vi "Calculadora con todo.vi"() -> ()   [LabVIEW 2020]
panel:
  in  "stop":bool
  in  "FUNCIONES":T1(ring)
  out "RESULTADO":dbl
  in  "NUM 2":dbl
  in  "NUM 1":dbl
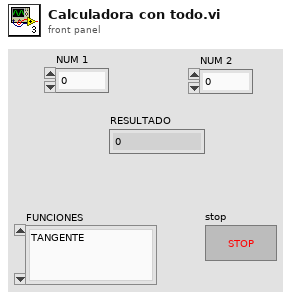
[diagram p1: front panel]
types:
  T1 = enum16{"TANGENTE", "COSENO", "SENO", "EXPONENCIAL", "CONVERSION GRADOS A RADIANES", "RAIZ CUADRADA", "DIVISION", "MULTIPLICACION", "RESTA", "SUMA"}
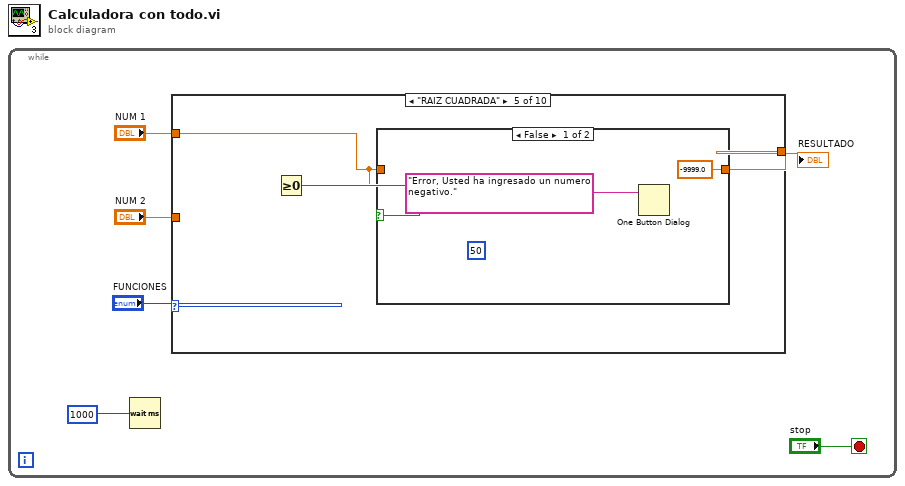
[diagram p0: block diagram]
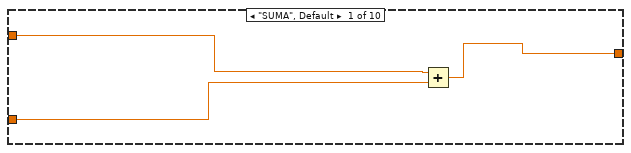
[diagram p2: hidden frame]
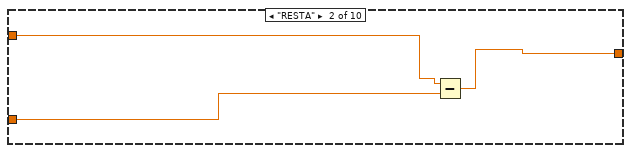
[diagram p3: hidden frame]
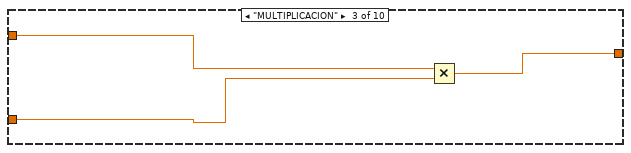
[diagram p4: hidden frame]
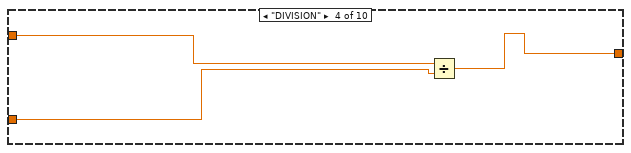
[diagram p5: hidden frame]
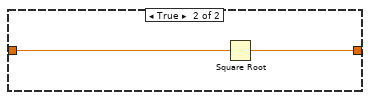
[diagram p6: hidden frame]
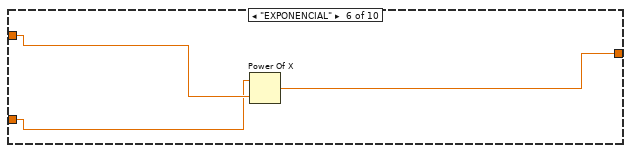
[diagram p7: hidden frame]
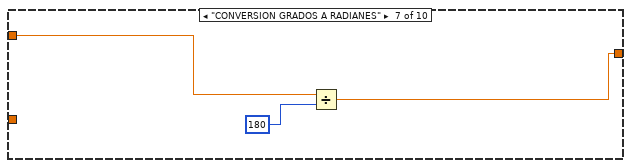
[diagram p8: hidden frame]
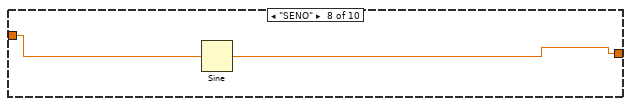
[diagram p9: hidden frame]
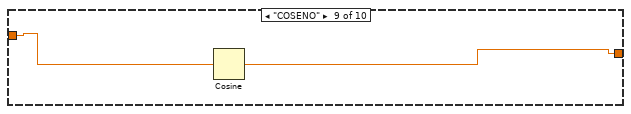
[diagram p10: hidden frame]
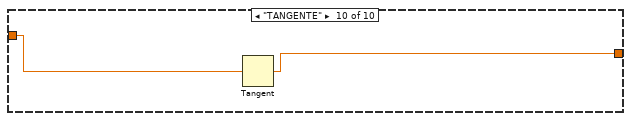
[diagram p11: hidden frame]
diagram:
  n1 = while {
    stop <- "stop" stop-if-true
    n2 = Wait (ms)(milliseconds to wait=1000) -> ()  [unwired: 1 out]
    n3 = case shown="\"RAIZ CUADRADA\"" "FUNCIONES" {
      tunnel: "NUM 1" -> [w9 w12 w15 w18 w19 w27 w29 w33 w35 w37]
      tunnel: "NUM 2" -> [w8 w11 w14 w17 _ w26 _ _ _ _]
      tunnel: [w7 w10 w13 w16 w20 w28 w30 w32 w34 w36] -> w4
      frame "SUMA", Default {
        n4 = Add(x=w9, y=w8) -> (x+y=w7:dbl)
      }
      frame "RESTA" {
        n5 = Subtract(x=w12, y=w11) -> (x-y=w10:dbl)
      }
      frame "MULTIPLICACION" {
        n6 = Multiply(x=w15, y=w14) -> (x*y=w13:dbl)
      }
      frame "DIVISION" {
        n7 = Divide(x=w18, y=w17) -> (x/y=w16:dbl)
      }
      frame "RAIZ CUADRADA" {
        n8 = Greater Or Equal To 0?(x=w19) -> (x >= 0?=w21:bool)
        n9 = case shown="False" w21 {
          tunnel: [-9999.0 w25] -> w20
          tunnel: w19 -> [_ w24]
          frame False {
            (unwired) 50
            n10 = One Button Dialog(message="Error, Usted ha ingresado un numero negativo.") -> ()  [unwired: 1 in, 1 out]
          }
          frame True {
            n11 = Square Root(x=w24) -> (sqrt(x)=w25:dbl)
          }
        }
      }
      frame "EXPONENCIAL" {
        n12 = Power Of X(1:w27, 2:w26) -> (0:w28:dbl)
      }
      frame "CONVERSION GRADOS A RADIANES" {
        n13 = Divide(x=w29, y=180) -> (x/y=w30:dbl)
      }
      frame "SENO" {
        n14 = Sine(x=w33) -> (sin(x)=w32:dbl)
      }
      frame "COSENO" {
        n15 = Cosine(x=w35) -> (cos(x)=w34:dbl)
      }
      frame "TANGENTE" {
        n16 = Tangent(1:w37) -> (0:w36:dbl)
      }
    }
    "RESULTADO" <- w4
  }
